vi "write_notifiers_to_string.vi"(7 "QueueRef":T1, 10 "Mission Notifiers":T3, 11 "NotifierReff":T2) -> (3 "input cluster":cluster{"names":string, "value":variant})   [LabVIEW 2013]
doc: "Converts all notifiers to a string"
uses:
  Data/TypeDefs/MissionNotifiers.ctl
  Logic/Classes/Missions/GenericMission/GenericMission.lvclass
  Logic/Classes/Obstacle/Obstacle.lvclass
  Data/TypeDefs/Notifiers.ctl
  Data/TypeDefs/UTM Location.ctl
  Data/TypeDefs/Sail Set Suggestions.ctl
  Data/TypeDefs/Rudder Set Suggestions.ctl
  Data/TypeDefs/OverrideInformation.ctl
  Data/TypeDefs/OverrideMode.ctl
  Data/TypeDefs/MotorSetup.ctl
  Data/TypeDefs/DynamixelSetupInfo.ctl
  Data/TypeDefs/AirmarStatus.ctl
  Data/TypeDefs/HardwareOnline.ctl
  Data/TypeDefs/DynamixelCycleTracker.ctl
  Data/TypeDefs/RC Input Values.ctl
  Logic/Classes/Waypoint/Waypoint.lvclass
  Data/TypeDefs/Queues.ctl
  Data/TypeDefs/Log_Data.ctl
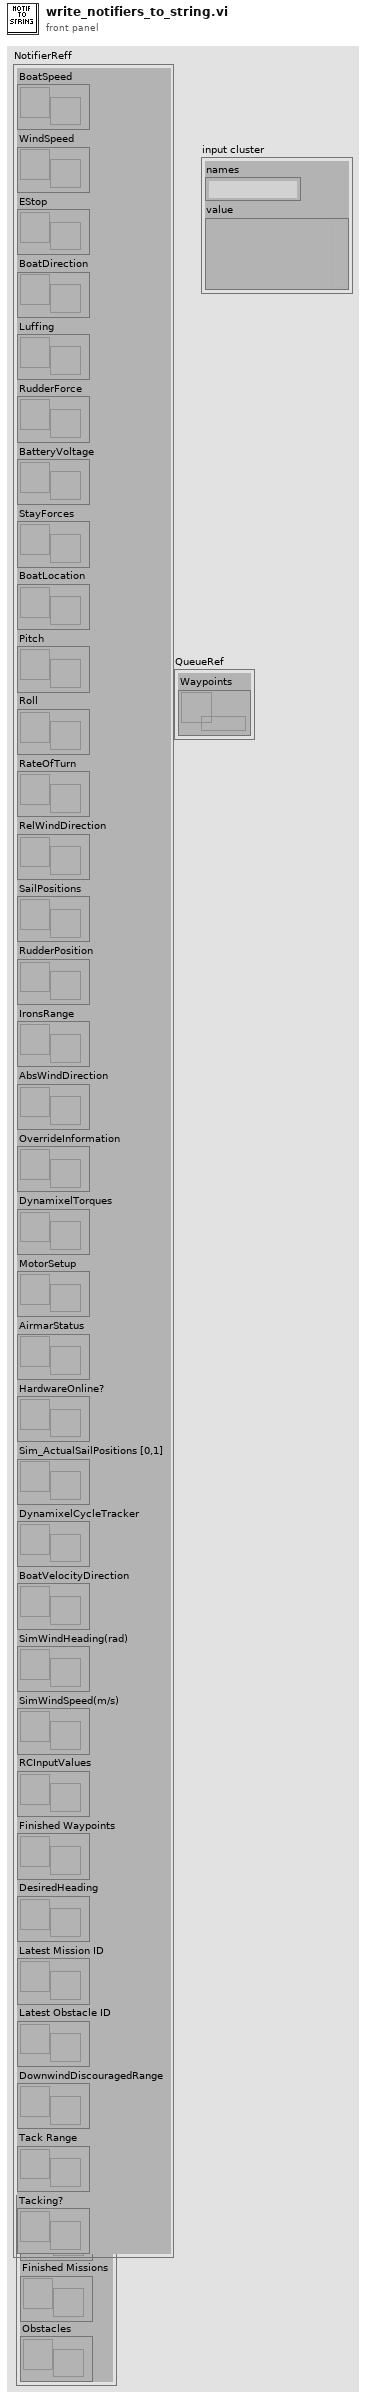
[diagram p1: front panel]
types:
  T1 = typedef "Queues.ctl" = cluster{"Waypoints":refnum<queue>}
  T2 = typedef "Notifiers.ctl" = cluster{"BoatSpeed":refnum<notifier>, "WindSpeed":refnum<notifier>, "EStop":refnum<notifier>, "BoatDirection":refnum<notifier>, "Luffing":refnum<notifier>, "RudderForce":refnum<notifier>, "BatteryVoltage":refnum<notifier>, "StayForces":refnum<notifier>, "BoatLocation":refnum<notifier>, "Pitch":refnum<notifier>, "Roll":refnum<notifier>, "RateOfTurn":refnum<notifier>, "RelWindDirection":refnum<notifier>, "SailPositions":refnum<notifier>, "RudderPosition":refnum<notifier>, "IronsRange":refnum<notifier>, "AbsWindDirection":refnum<notifier>, "OverrideInformation":refnum<notifier>, "DynamixelTorques":refnum<notifier>, "MotorSetup":refnum<notifier>, "AirmarStatus":refnum<notifier>, "HardwareOnline?":refnum<notifier>, "Sim_ActualSailPositions [0,1]":refnum<notifier>, "DynamixelCycleTracker":refnum<notifier>, "BoatVelocityDirection":refnum<notifier>, "SimWindHeading(rad)":refnum<notifier>, "SimWindSpeed(m/s)":refnum<notifier>, "RCInputValues":refnum<notifier>, "Finished Waypoints":refnum<notifier>, "DesiredHeading":refnum<notifier>, "Latest Mission ID":refnum<notifier>, "Latest Obstacle ID":refnum<notifier>, "DownwindDiscouragedRange":refnum<notifier>, "Tack Range":refnum<notifier>, "Tacking?":refnum<notifier>}
  T3 = typedef "MissionNotifiers.ctl" = cluster{"Missions":refnum<notifier>, "Finished Missions":refnum<notifier>, "Obstacles":refnum<notifier>}
  T4 = typedef "Log_Data.ctl" = cluster{"names":string, "value":variant}
  T5 = typedef "HardwareOnline.ctl" = cluster{"AirmarOnline":bool, "WindvaneOnline":bool, "HemisphereOnline":bool, "StayForceOnline":bool, "BatteryVoltageOnline":bool, "AccelerometerOnline":bool, "MainDynamixel Online":bool, "JibDynamixel Online":bool, "RudderDynamixel Online":bool}
  T6 = typedef "MotorSetup.ctl" = cluster{"Main Dynamixel Set Data":T7, "Rudder Dynamixel Set Data":T7, "Jib Dynamixel Set Data":T7}
  T7 = typedef "DynamixelSetupInfo.ctl" = cluster{"Lower Winch Bound (deg)":dbl, "Upper Winch Bound (deg)":dbl}
  T8 = typedef "OverrideInformation.ctl" = cluster{"OverrideMode":T9, "SailSetting":T10, "Rudder Setpoint":T11, "Sim_Wind_Speed":dbl, "Sim_Wind_Heading":dbl}
  T9 = typedef "OverrideMode.ctl" = enum16{"None", "Rudder", "Sails", "Both"}
  T10 = typedef "Sail Set Suggestions.ctl" = cluster{"MainSailSuggestion":dbl, "JibSailSuggestion":dbl}
  T11 = typedef "Rudder Set Suggestions.ctl" = dbl
  T12 = typedef "UTM Location.ctl" = cluster{"UTM Zone":dbl, "Hemisphere":enum16{"North", "South"}, "East":dbl, "North":dbl}
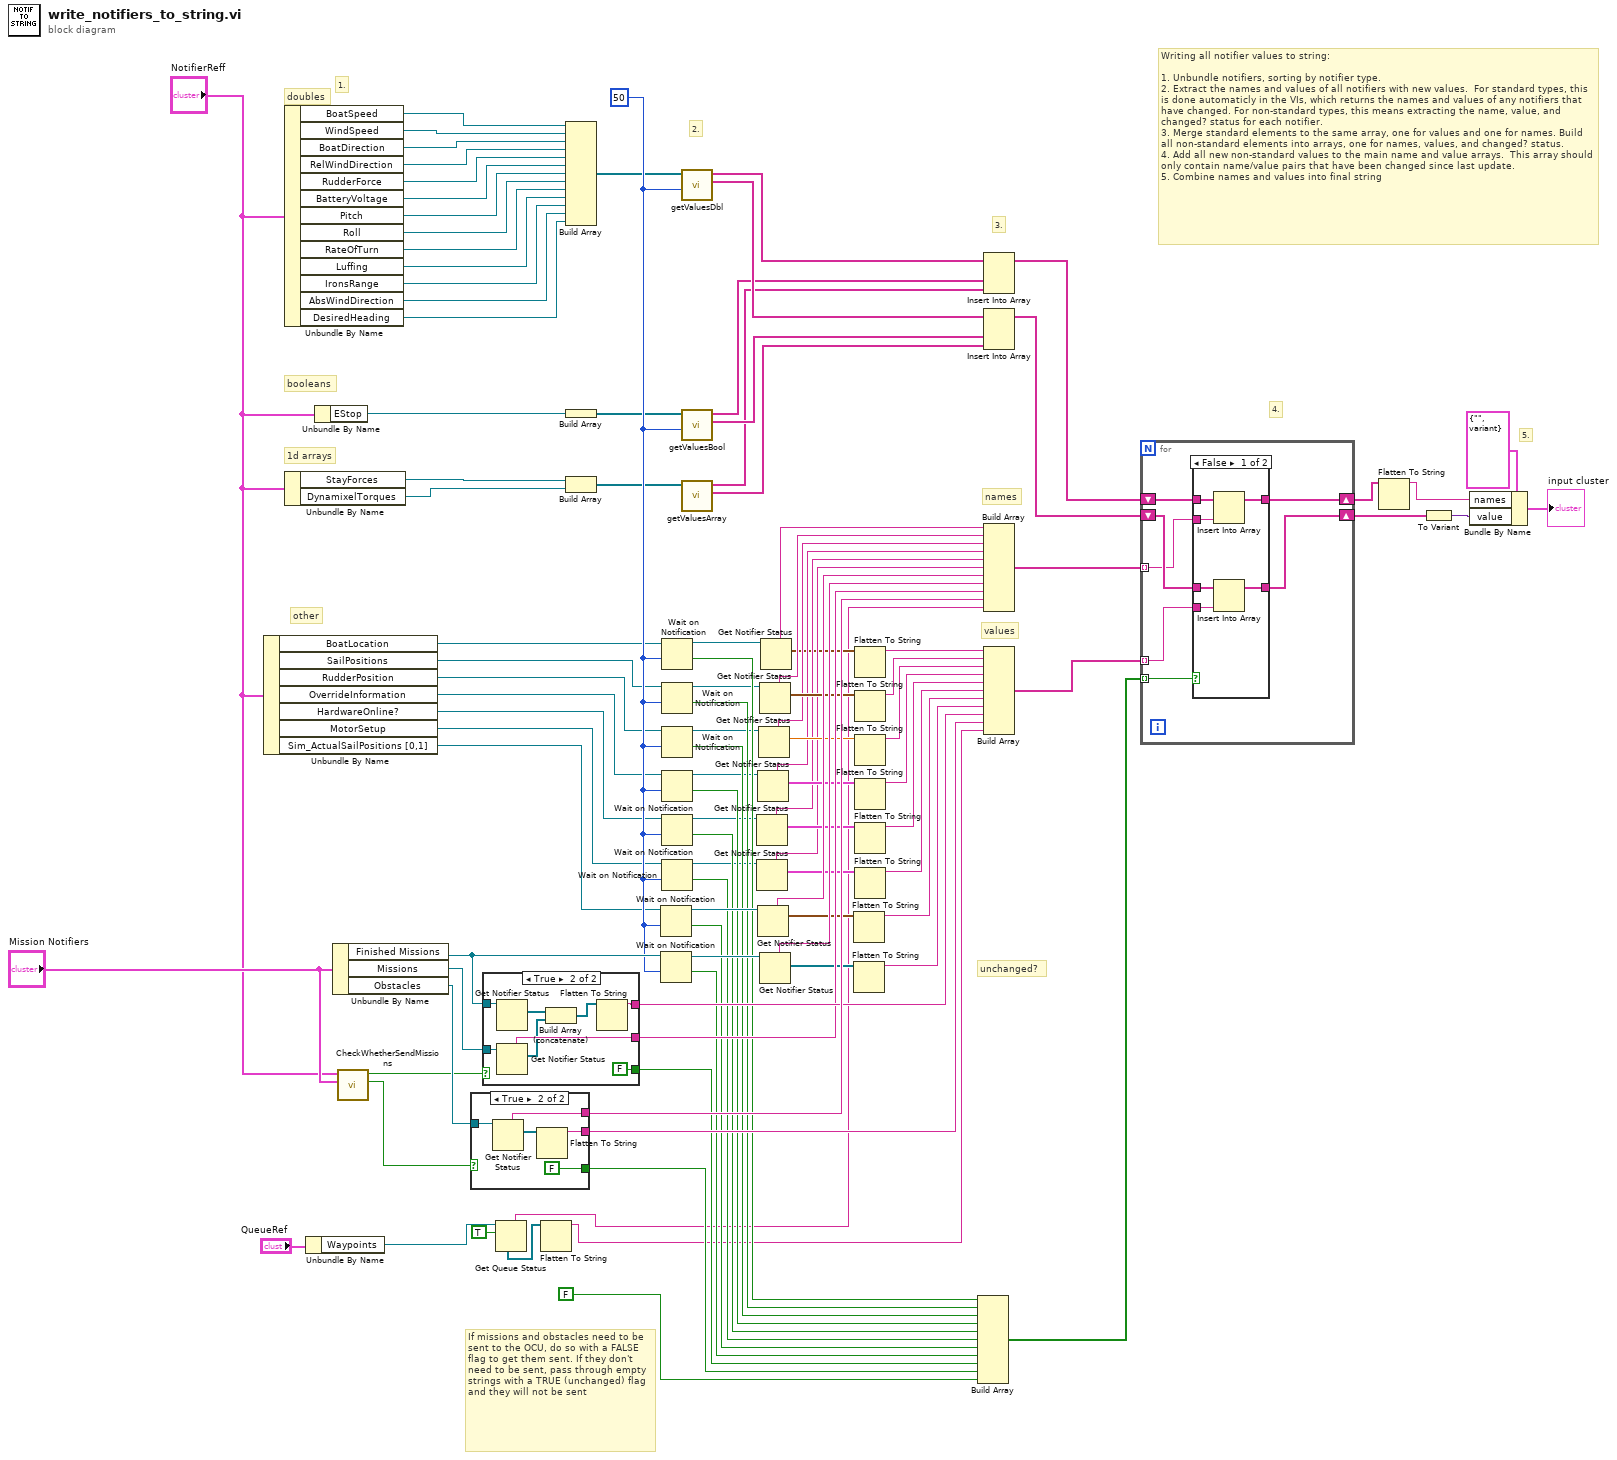
[diagram p0: block diagram]
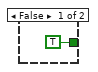
[diagram p2: hidden frame]
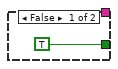
[diagram p3: hidden frame]
diagram:
  w92 = 50 ("timeout in ms (-1)")
  # "5."
  # "If missions and obstacles need to be sent to the OCU, do so with a FALSE flag to get them sent. If they don't need to be sent, pass through empty strings with a TRUE (unchanged) flag and they will not be sent"
  # "Writing all notifier values to string:\n\n1. Unbundle notifiers, sorting by notifier type.\n2. Extract the names and values of all notifiers with new values.  For standard types, this is done automaticly in the VIs, which returns the names and values of any notifiers that have changed. For non-standard types, this means extracting the name, value, and changed? status for each notifier. \n3. Merge standard elements to the same array, one for values and one for names. Build all non-standard elements into arrays, one for names, values, and changed? status.\n4. Add all new non-standard values to the main name and value arrays.  This array should only contain name/value pairs that have been changed since last update.\n5. Combine names and values into final string"
  # "4."
  # "3."
  # "2."
  # "1."
  # "unchanged?"
  # "values"
  # "names"
  # "other"
  # "1d arrays"
  # "booleans"
  # "doubles"
  n1 = Unbundle By Name("NotifierReff") -> ("BoatLocation"=w22:refnum<notifier>, "SailPositions"=w23:refnum<notifier>, "RudderPosition"=w24:refnum<notifier>, "OverrideInformation"=w26:refnum<notifier>, "HardwareOnline?"=w25:refnum<notifier>, "MotorSetup"=w27:refnum<notifier>, "Sim_ActualSailPositions [0,1]"=w78:refnum<notifier>)
  n2 = Unbundle By Name("NotifierReff") -> ("BoatSpeed"=w91:refnum<notifier>, "WindSpeed"=w90:refnum<notifier>, "BoatDirection"=w10:refnum<notifier>, "RelWindDirection"=w93:refnum<notifier>, "RudderForce"=w11:refnum<notifier>, "BatteryVoltage"=w12:refnum<notifier>, "Pitch"=w13:refnum<notifier>, "Roll"=w14:refnum<notifier>, "RateOfTurn"=w15:refnum<notifier>, "Luffing"=w16:refnum<notifier>, "IronsRange"=w17:refnum<notifier>, "AbsWindDirection"=w18:refnum<notifier>, "DesiredHeading"=w89:refnum<notifier>)
  n3 = Unbundle By Name("NotifierReff") -> ("StayForces"=w21:refnum<notifier>, "DynamixelTorques"=w20:refnum<notifier>)
  n4 = Unbundle By Name("QueueRef") -> ("Waypoints"=w7:refnum<queue>)
  n5 = Unbundle By Name("NotifierReff") -> ("EStop"=w19:refnum<notifier>)
  n6 = Unbundle By Name("Mission Notifiers") -> ("Finished Missions"=w104:refnum<notifier>, "Missions"=w96:refnum<notifier>, "Obstacles"=w100:refnum<notifier>)
  n7 = call "CheckWhetherSendMissions.vi"("Mission Notifiers"="Mission Notifiers", "NotifierReff"="NotifierReff") -> ("Send obstacles?"=w101:bool, "Send missions?"=w6:bool)  [unwired: 8 in]
  n8 = case shown="True" w101 {
    tunnel: w100 -> [_ w110]
    tunnel: [_ w109] -> w102
    tunnel: [_ w107] -> w103
    tunnel: [TRUE FALSE] -> w8
    frame False {
    }
    frame True {
      n9 = Get Notifier Status(notifier=w110) -> (notifier name=w109:string, current notification=w108:refnum<class "Obstacle.lvclass">[])  [unwired: 1 in, 3 out]
      n10 = Flatten To String(anything=w108) -> (data string=w107:string)  [unwired: 3 in, 2 out]
    }
  }
  n11 = case shown="True" w6 {
    tunnel: w96 -> [_ w117]
    tunnel: [_ w115] -> w97
    tunnel: [_ w119] -> w98
    tunnel: [TRUE FALSE] -> w99
    tunnel: w104 -> [_ w116]
    frame False {
    }
    frame True {
      n12 = Get Notifier Status(notifier=w116) -> (current notification=w114:refnum<class "GenericMission.lvclass">[])  [unwired: 1 in, 4 out]
      n13 = Get Notifier Status(notifier=w117) -> (notifier name=w115:string, current notification=w112:refnum<class "GenericMission.lvclass">[])  [unwired: 1 in, 3 out]
      n14 = Build Array (concatenate)(w114, w112) -> (w113:refnum<class "GenericMission.lvclass">[])
      n15 = Flatten To String(anything=w113) -> (data string=w119:string)  [unwired: 3 in, 2 out]
    }
  }
  n16 = Get Queue Status(queue=w7, return elements? (F)=TRUE) -> (queue name=w5:string, elements=w2:refnum<class "Waypoint.lvclass">[])  [unwired: 1 in, 6 out]
  n17 = Flatten To String(anything=w2) -> (data string=w4:string)  [unwired: 3 in, 2 out]
  n18 = Build Array(w91, w90, w10, w93, w11, w12, w13, w14, w15, w16, w17, w18, w89) -> (w34:refnum<notifier>[])
  n19 = Build Array(w19) -> (w35:refnum<notifier>[])
  n20 = Build Array(w21, w20) -> (w36:refnum<notifier>[])
  n21 = Wait on Notification(notifier=w78, timeout in ms (-1)=w92) -> (notifier out=w79:refnum<notifier>, timed out?=w83:bool)  [unwired: 2 in, 2 out]
  n22 = Wait on Notification(notifier=w104, timeout in ms (-1)=w92) -> (notifier out=w85:refnum<notifier>, timed out?=w84:bool)  [unwired: 2 in, 2 out]
  n23 = Wait on Notification(notifier=w22, timeout in ms (-1)=w92) -> (notifier out=w37:refnum<notifier>, timed out?=w60:bool)  [unwired: 2 in, 2 out]
  n24 = Wait on Notification(notifier=w23, timeout in ms (-1)=w92) -> (notifier out=w40:refnum<notifier>, timed out?=w59:bool)  [unwired: 2 in, 2 out]
  n25 = Wait on Notification(notifier=w24, timeout in ms (-1)=w92) -> (notifier out=w42:refnum<notifier>, timed out?=w58:bool)  [unwired: 2 in, 2 out]
  n26 = Wait on Notification(notifier=w26, timeout in ms (-1)=w92) -> (notifier out=w44:refnum<notifier>, timed out?=w57:bool)  [unwired: 2 in, 2 out]
  n27 = Wait on Notification(notifier=w25, timeout in ms (-1)=w92) -> (notifier out=w46:refnum<notifier>, timed out?=w56:bool)  [unwired: 2 in, 2 out]
  n28 = Wait on Notification(notifier=w27, timeout in ms (-1)=w92) -> (notifier out=w48:refnum<notifier>, timed out?=w55:bool)  [unwired: 2 in, 2 out]
  n29 = call "getValuesDbl.vi"("timeout in ms (-1)"=w92, "notifiers in"=w34) -> ("notifier values"=w64:string[], "notifier names"=w61:string[])  [unwired: 7 in, 1 out]
  n30 = call "getValuesBool.vi"("timeout in ms (-1)"=w92, "notifiers in"=w35) -> ("notifier values"=w65:string[], "notifier names"=w62:string[])  [unwired: 7 in, 1 out]
  n31 = call "getValuesArray.vi"("appended array"=w36) -> ("notifier values"=w66:string[], "notifier names"=w63:string[])  [unwired: 8 in, 1 out]
  n32 = Get Notifier Status(notifier=w46) -> (notifier name=w47:string, current notification=w53:T5)  [unwired: 1 in, 3 out]
  n33 = Get Notifier Status(notifier=w48) -> (notifier name=w49:string, current notification=w54:T6)  [unwired: 1 in, 3 out]
  n34 = Get Notifier Status(notifier=w44) -> (notifier name=w45:string, current notification=w52:T8)  [unwired: 1 in, 3 out]
  n35 = Get Notifier Status(notifier=w79) -> (notifier name=w82:string, current notification=w80:T10)  [unwired: 1 in, 3 out]
  n36 = Get Notifier Status(notifier=w42) -> (notifier name=w43:string, current notification=w51:T11)  [unwired: 1 in, 3 out]
  n37 = Get Notifier Status(notifier=w40) -> (notifier name=w41:string, current notification=w50:T10)  [unwired: 1 in, 3 out]
  n38 = Get Notifier Status(notifier=w85) -> (notifier name=w86:string, current notification=w87:refnum<class "GenericMission.lvclass">[])  [unwired: 1 in, 3 out]
  n39 = Get Notifier Status(notifier=w37) -> (notifier name=w39:string, current notification=w38:T12)  [unwired: 1 in, 3 out]
  n40 = Flatten To String(anything=w80) -> (data string=w81:string)  [unwired: 3 in, 2 out]
  n41 = Flatten To String(anything=w87) -> (data string=w88:string)  [unwired: 3 in, 2 out]
  n42 = Flatten To String(anything=w38) -> (data string=w28:string)  [unwired: 3 in, 2 out]
  n43 = Flatten To String(anything=w50) -> (data string=w29:string)  [unwired: 3 in, 2 out]
  n44 = Flatten To String(anything=w51) -> (data string=w30:string)  [unwired: 3 in, 2 out]
  n45 = Flatten To String(anything=w52) -> (data string=w31:string)  [unwired: 3 in, 2 out]
  n46 = Flatten To String(anything=w53) -> (data string=w32:string)  [unwired: 3 in, 2 out]
  n47 = Flatten To String(anything=w54) -> (data string=w33:string)  [unwired: 3 in, 2 out]
  n48 = Build Array(w60, w59, w58, w57, w56, w55, w83, w84, w99, w8, FALSE) -> (w69:bool[])
  n49 = Insert Into Array(array=w61, new element #1=w62, new element #2=w63) -> (w67:string[])  [unwired: 1 in]
  n50 = Insert Into Array(array=w64, new element #1=w65, new element #2=w66) -> (w68:string[])  [unwired: 1 in]
  n51 = Build Array(w39, w41, w43, w45, w47, w49, w82, w86, w97, w102, w5) -> (w70:string[])
  n52 = Build Array(w28, w29, w30, w31, w32, w33, w81, w88, w98, w103, w4) -> (w71:string[])
  n53 = for {
    tunnel: w69 -> [w126] mode=indexing
    shift-right: [w125] -> w76
    shift-left: w67 -> [w120]
    shift-right: [w123] -> w72
    shift-left: w68 -> [w124]
    tunnel: w70 -> [w122] mode=indexing
    tunnel: w71 -> [w121] mode=indexing
    n54 = case shown="False" w126 {
      tunnel: [w132 w133] -> w125
      tunnel: w124 -> [w131 w134]
      tunnel: [w130 w134] -> w123
      tunnel: w122 -> [w129 _]
      tunnel: w121 -> [w128 _]
      tunnel: w120 -> [w127 w133]
      frame False {
        n55 = Insert Into Array(array=w127, new element=w129) -> (w132:string[])  [unwired: 1 in]
        n56 = Insert Into Array(array=w131, new element=w128) -> (w130:string[])  [unwired: 1 in]
      }
      frame True {
      }
    }
  }
  n57 = Flatten To String(anything=w76) -> (data string=w77:string)  [unwired: 3 in, 2 out]
  n58 = To Variant(anything=w72) -> (Variant=w75:variant)
  n59 = Bundle By Name(cluster=T4 {"names"="", "value"=variant} ("input cluster"), "names"=w77, "value"=w75) -> (→"input cluster":T4)
